vi "Distance Between Gates - Constant.vi"() -> (3 "Distance Between Gates (m)":dbl)   [LabVIEW 2020]
doc: "The distance (meters) between the two optical gates which measure the speed of the projectile."
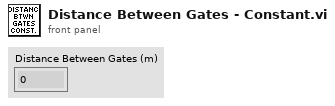
[diagram p1: front panel]
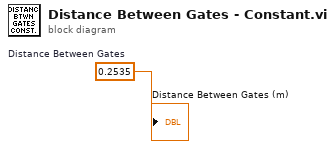
[diagram p0: block diagram]
diagram:
  w1 = 0.2535  # Distance Between Gates
  "Distance Between Gates (m)" <- w1
